vi "Add New Children.vi"(8 "error in (no error)":errorcluster, 9 "Folder Names":string[](array[string]), 10 "Parent Tag":string, 11 "Tree In":refnum<vi>) -> (0 "error out":errorcluster, 1 "Folder Names Dup":string[](array[string]), 2 "Parent Tag Dup":string, 3 "Tree Out":refnum<vi>)   [LabVIEW 2018, in "Tree Browser.lvlib"]
doc: "Adds new children under a parent node which exist on disk but not in the tree."
uses:
  Tree Browser.lvlib
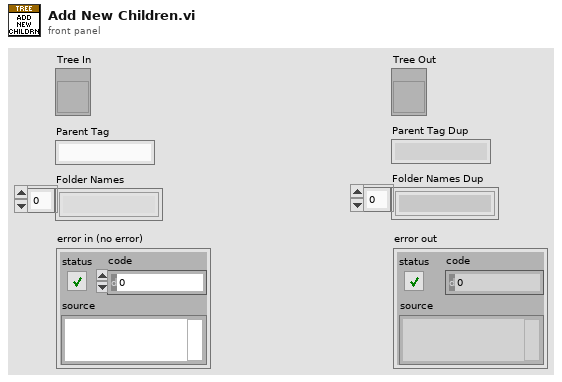
[diagram p1: front panel]
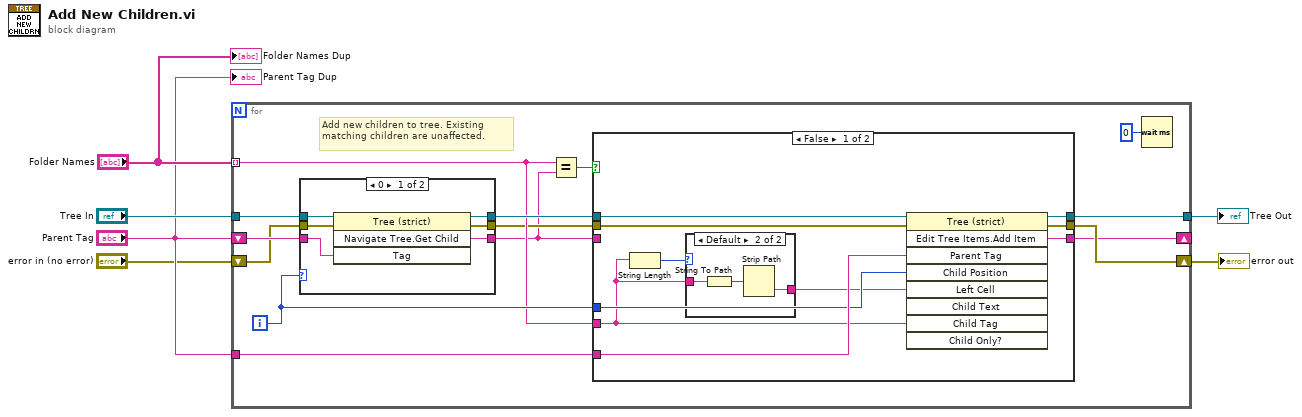
[diagram p0: block diagram]
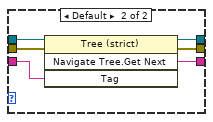
[diagram p4: hidden frame]
diagram:
  n1 = for {
    tunnel: "Tree In" -> [w20]
    shift-right: [w9] -> _
    shift-left: "Parent Tag" -> [w19]
    tunnel: "Folder Names" -> [w15] mode=indexing
    tunnel: "Parent Tag" -> [w18]
    tunnel: [w13] -> w4
    shift-right: [w10] -> w1
    shift-left: "error in (no error)" -> [w12]
    i -> [w16]
    # "Add new children to tree. Existing matching children are unaffected."
    n2 = case shown="0" w16 {
      tunnel: w20 -> [w43 w49]
      tunnel: w19 -> [w42 w48]
      tunnel: [w41 w47] -> w8
      tunnel: [w40 w46] -> w17
      tunnel: w12 -> [w39 w45]
      tunnel: [w38 w44] -> w11
      frame 0 {
        n3 = invoke class="Tree (strict)" method="Navigate Tree.Get Child"(reference=w43, error in=w39, "Tag"=w42) -> (reference out=w40:refnum<vi>, error out=w38:errorcluster, "Navigate Tree:Get Child"=w41:string)  [unwired: 1 in, 1 out]
      }
      frame Default {
        n4 = invoke class="Tree (strict)" method="Navigate Tree.Get Next"(reference=w49, error in=w45, "Tag"=w48) -> (reference out=w46:refnum<vi>, error out=w44:errorcluster, "Navigate Tree:Get Next Item"=w47:string)  [unwired: 1 in, 1 out]
      }
    }
    n5 = Equal?(x=w15, y=w8) -> (x = y?=w14:bool)
    n6 = case shown="False" w14 {
      tunnel: w18 -> [w30 _]
      tunnel: w17 -> [w29 w37]
      tunnel: w16 -> [w28 _]
      tunnel: w15 -> [w22 _]
      tunnel: [w27 w37] -> w13
      tunnel: w11 -> [w26 w36]
      tunnel: [w25 w36] -> w10
      tunnel: [w23 w35] -> w9
      tunnel: w8 -> [_ w35]
      frame False {
        n7 = String Length(string=w22) -> (length=w21:i32)
        n8 = case shown="Default" w21 {
          tunnel: w22 -> [w31 w34]
          tunnel: [w31 w32] -> w24
          frame 3 {
          }
          frame Default {
            n9 = String To Path(string=w34) -> (path=w33:path)
            n10 = Strip Path(path=w33) -> (name=w32:string)  [unwired: 1 out]
          }
        }
        n11 = invoke class="Tree (strict)" method="Edit Tree Items.Add Item"(reference=w29, error in=w26, "Parent Tag"=w30, "Child Position"=w28, "Left Cell"=w24, "Child Tag"=w22) -> (reference out=w27:refnum<vi>, error out=w25:errorcluster, "Edit Tree Items:Add Item"=w23:string)  [unwired: 3 in, 6 out]
      }
      frame True {
      }
    }
    n12 = Wait (ms)(milliseconds to wait=u32 0) -> ()  [unwired: 1 out]
  }
  "Tree Out" <- w4
  "error out" <- w1
  "Parent Tag Dup" <- "Parent Tag"
  "Folder Names Dup" <- "Folder Names"
